vi "LuaVIEW Compile Execute Call.vi"() -> (0 "pass?":bool)   [LabVIEW 2012]
uses:
  typedefs/t_LuaVIEW Reference.ctl
  typedefs/t_LuaVIEW CIN Spinlocked Actions.ctl
  subvis/private/LuaVIEW Pull (string).vi
  subvis/private/LuaVIEW Push (I32).vi
  subvis/private/LuaVIEW Pull (number).vi
  subvis/private/LuaVIEW Push (number).vi
  subvis/private/LuaVIEW Pull (I32).vi
panel:
  in  "script file":path=path "scripts/compile execute call.lua"
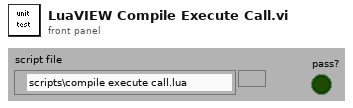
[diagram p1: front panel]
types:
  T1 = enum32{"execute", "initialize", "open_base_state([str:ident])", "open_private_state()", "I32:num=open_states()", "compile(str:name,str:script)", "execute()", "[num:res],...=call(str:function,[num:arg],...)", "[num:res],...=call_required(str:function,I32:required,[num:arg],...)", "close()", "cleanup"}
  T2 = typedef "t_LuaVIEW CIN Spinlocked Actions.ctl" = enum16{"totals", "taskcount", "open", "registerpublic", "registerexport", "revokeexports", "unregnextpublic", "usepublic", "pollexport", "close", "startyieldtest", "endyieldtest", "pollprintbuffer"}
  T3 = typedef "t_LuaVIEW Reference.ctl" = refnum<k1>
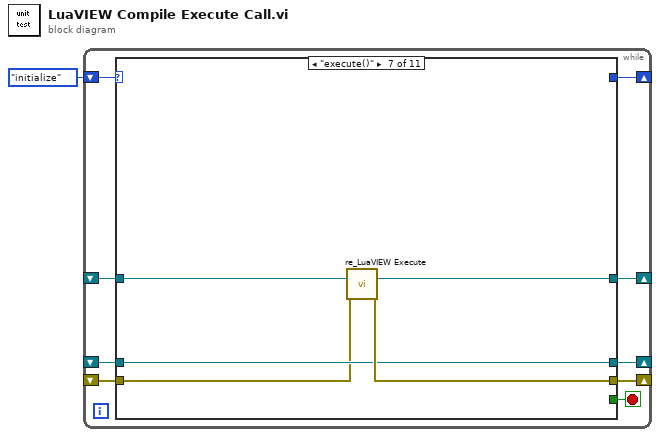
[diagram p0: block diagram]
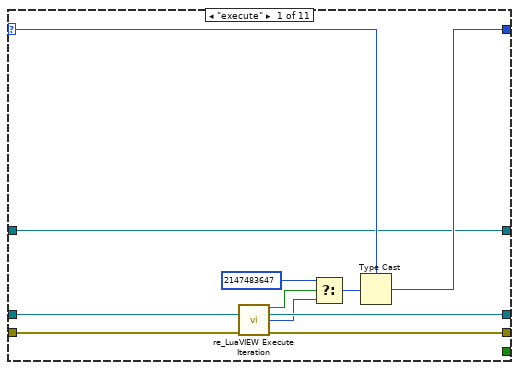
[diagram p2: hidden frame]
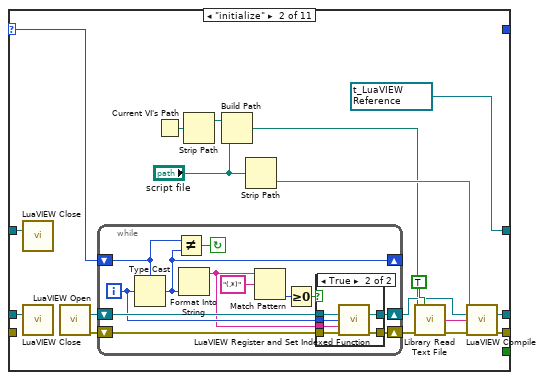
[diagram p3: hidden frame]
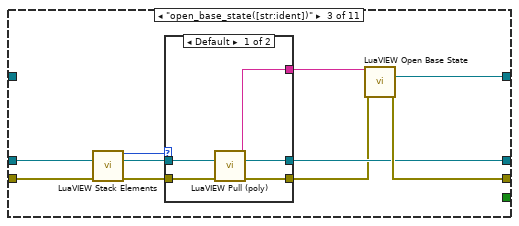
[diagram p5: hidden frame]
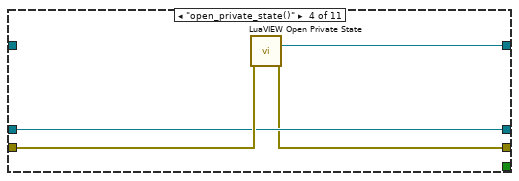
[diagram p7: hidden frame]
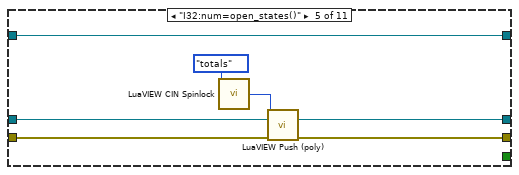
[diagram p8: hidden frame]
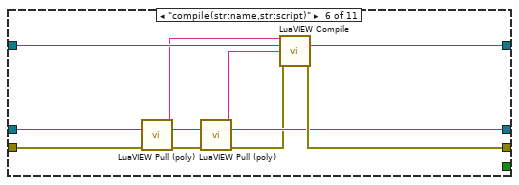
[diagram p9: hidden frame]
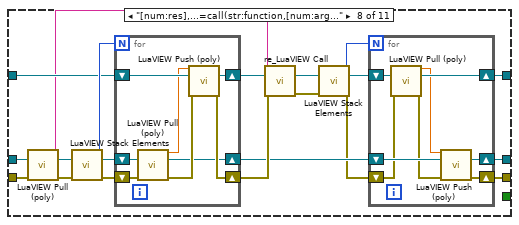
[diagram p10: hidden frame]
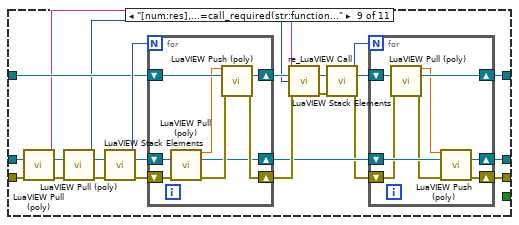
[diagram p11: hidden frame]
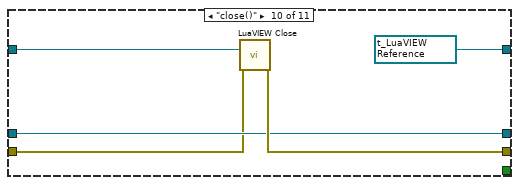
[diagram p12: hidden frame]
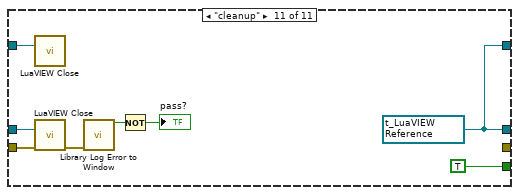
[diagram p13: hidden frame]
diagram:
  n1 = while {
    shift-right: [w8] -> _
    shift-left: T1."initialize" -> [w10]
    shift-right: [w6] -> _
    shift-left: _ -> [w7]
    shift-right: [w5] -> _
    shift-left: _ -> [w4]
    shift-right: [w3] -> _
    shift-left: _ -> [w2]
    stop <- w9 stop-if-true
    n2 = case shown="\"execute()\"" w10 {
      selector: w10 -> [w14 w35 _ _ _ _ _ _ _ _ _]
      tunnel: [_ _ _ _ _ _ _ _ _ _ TRUE] -> w9
      tunnel: [w12 _ _ _ _ _ _ _ _ _ _] -> w8
      tunnel: w7 -> [w21 w39 w66 w79 w81 w91 w100 w115 w156 w181 w191]
      tunnel: [w18 w36 w63 w79 w82 w95 w100 w105 w146 w181 w184] -> w6
      tunnel: [w19 w34 w69 w78 w83 w98 w103 w106 w147 w183 _] -> w5
      tunnel: w4 -> [w20 _ w67 w80 w85 w90 w99 w116 w157 w180 w189]
      tunnel: [w11 w22 w68 w77 w87 w97 w102 w104 w145 w179 w184] -> w3
      tunnel: w2 -> [w11 w23 _ _ w87 w96 w101 w120 w159 w182 w185]
      frame "execute" {
        n3 = call "re_LuaVIEW Execute Iteration.vi"("LuaVIEW reference in"=w21, "init or indexed function error"=w20) -> ("last?"=w16:bool, "LuaVIEW reference out"=w18:T3, "function index"=w17:i32, "final error"=w19:errorcluster)  [unwired: 10 in]
        n4 = Select(t=2147483647, s=w16, f=w17) -> (s? t:f=w13:i32)
        n5 = Type Cast(type=w14, x=w13) -> (*(type *) &x=w12:T1)
      }
      frame "initialize" {
        w22 = T3 refnum items=["LuaVIEW"] ("LuaVIEW reference")
        n6 = call "LuaVIEW Close.vi"("LuaVIEW reference"=w23) -> ()  [unwired: 14 in, 1 out]
        n7 = call "LuaVIEW Close.vi"("LuaVIEW reference"=w39) -> ()  [unwired: 14 in, 1 out]
        n8 = call "LuaVIEW Open.vi"() -> ("LuaVIEW reference"=w37:T3, "error out"=w38:errorcluster)  [unwired: 14 in]
        n9 = while {
          shift-right: [w45] -> w30
          shift-left: w38 -> [w48]
          shift-right: [w46] -> w31
          shift-left: w37 -> [w47]
          shift-right: [w40] -> _
          shift-left: w35 -> [w41]
          i -> [w44]
          stop <- w51 continue-if-true
          n10 = Type Cast(type=w41, x=w44) -> (*(type *) &x=w40:T1)
          n11 = Not Equal?(x=w41, y=w40) -> (x != y?=w51:bool)
          n12 = Format Into String(w40) -> (resulting string=w42:string)  [unwired: 3 in, 1 out]
          n13 = Match Pattern(string=w42, regular expression="(.*)") -> (offset past match=w49:i32)  [unwired: 1 in, 3 out]
          n14 = Greater Or Equal To 0?(x=w49) -> (x >= 0?=w43:bool)
          n15 = case shown="True" w43 {
            tunnel: w47 -> [w53 w56]
            tunnel: w44 -> [_ w57]
            tunnel: w42 -> [_ w54]
            tunnel: [w52 w59] -> w45
            tunnel: [w53 w58] -> w46
            tunnel: w48 -> [w52 w55]
            frame False {
            }
            frame True {
              n16 = call "LuaVIEW Register and Set Indexed Function.vi"("LuaVIEW reference in"=w56, "index"=w57, "synopsis"=w54, "error in (no error)"=w55) -> ("LuaVIEW reference out"=w58:T3, "error out"=w59:errorcluster)  [unwired: 10 in]
            }
          }
        }
        n17 = Current VI's Path() -> (path=w28:path)
        n18 = Strip Path(path=w28) -> (stripped path=w27:path)  [unwired: 1 out]
        n19 = Build Path(base path=w27, name or relative path="script file") -> (appended path=w24:path)
        n20 = Strip Path(path="script file") -> (name=w25:string)  [unwired: 1 out]
        n21 = call "Library Read Text File.vi"("file path"=w24, "convert eol (F)"=TRUE, "error in (no error)"=w30) -> ("read text"=w29:string, "error out"=w32:errorcluster)  [unwired: 10 in, 1 out]
        n22 = call "LuaVIEW Compile.vi"("script name"=w25, "LuaVIEW reference in"=w31, "script"=w29, "error in (no error)"=w32) -> ("LuaVIEW reference out"=w36:T3, "error out"=w34:errorcluster)  [unwired: 10 in]
      }
      frame "open_base_state([str:ident])" {
        n23 = call "LuaVIEW Stack Elements.vi"("LuaVIEW reference in"=w66, "error in (no error)"=w67) -> ("elements"=w65:i32, "LuaVIEW reference out"=w64:T3, "error out"=w62:errorcluster)  [unwired: 11 in]
        n24 = case shown="Default" w65 {
          tunnel: [w71 w76] -> w63
          tunnel: w64 -> [w74 w76]
          tunnel: [w72 w75] -> w61
          tunnel: w62 -> [w73 w75]
          tunnel: [w70 _] -> w60
          frame Default {
            n25 = call-poly "LuaVIEW Pull (poly).vi"("LuaVIEW reference in"=w74, "error in (no error)"=w73) -> ("string"=w70:string, "LuaVIEW reference out"=w71:T3, "error out"=w72:errorcluster)  [unwired: 11 in]
          }
          frame 0 {
          }
        }
        n26 = call "LuaVIEW Open Base State.vi"("close identifier (none)"=w60, "error in (no error)"=w61) -> ("LuaVIEW reference"=w68:T3, "error out"=w69:errorcluster)  [unwired: 12 in]
      }
      frame "open_private_state()" {
        n27 = call "LuaVIEW Open Private State.vi"("error in (no error)"=w80) -> ("LuaVIEW reference"=w77:T3, "error out"=w78:errorcluster)  [unwired: 13 in]
      }
      frame "I32:num=open_states()" {
        n28 = call "LuaVIEW CIN Spinlock.vi"("action"=t_LuaVIEW_CIN_Spinlocked_Actions."totals") -> ("index out"=w84:i32)  [unwired: 8 in, 6 out]
        n29 = call-poly "LuaVIEW Push (poly).vi"("I32"=w84, "LuaVIEW reference in"=w81, "error in (no error)"=w85) -> ("LuaVIEW reference out"=w82:T3, "error out"=w83:errorcluster)  [unwired: 11 in]
      }
      frame "compile(str:name,str:script)" {
        n30 = call-poly "LuaVIEW Pull (poly).vi"("LuaVIEW reference in"=w91, "error in (no error)"=w90) -> ("string"=w88:string, "LuaVIEW reference out"=w93:T3, "error out"=w92:errorcluster)  [unwired: 11 in]
        n31 = call-poly "LuaVIEW Pull (poly).vi"("LuaVIEW reference in"=w93, "error in (no error)"=w92) -> ("string"=w89:string, "LuaVIEW reference out"=w95:T3, "error out"=w94:errorcluster)  [unwired: 11 in]
        n32 = call "LuaVIEW Compile.vi"("script name"=w88, "LuaVIEW reference in"=w96, "script"=w89, "error in (no error)"=w94) -> ("LuaVIEW reference out"=w97:T3, "error out"=w98:errorcluster)  [unwired: 10 in]
      }
      frame "execute()" {
        n33 = call "re_LuaVIEW Execute.vi"("LuaVIEW reference in"=w101, "error in (no error)"=w99) -> ("LuaVIEW reference out"=w102:T3, "error out"=w103:errorcluster)  [unwired: 12 in]
      }
      frame "[num:res],...=call(str:function,[num:arg],...)" {
        n34 = call-poly "LuaVIEW Pull (poly).vi"("LuaVIEW reference in"=w115, "error in (no error)"=w116) -> ("string"=w114:string, "LuaVIEW reference out"=w118:T3, "error out"=w117:errorcluster)  [unwired: 11 in]
        n35 = call "LuaVIEW Stack Elements.vi"("LuaVIEW reference in"=w118, "error in (no error)"=w117) -> ("elements"=w123:i32, "LuaVIEW reference out"=w121:T3, "error out"=w122:errorcluster)  [unwired: 11 in]
        n36 = for {
          N: w123 -> [_]
          shift-right: [w135] -> w113
          shift-left: w122 -> [w138]
          shift-right: [w134] -> w112
          shift-left: w121 -> [w139]
          shift-right: [w133] -> w119
          shift-left: w120 -> [w137]
          n37 = call-poly "LuaVIEW Pull (poly).vi"("LuaVIEW reference in"=w139, "error in (no error)"=w138) -> ("number"=w132:dbl, "LuaVIEW reference out"=w134:T3, "error out"=w136:errorcluster)  [unwired: 11 in]
          n38 = call-poly "LuaVIEW Push (poly).vi"("number"=w132, "LuaVIEW reference in"=w137, "error in (no error)"=w136) -> ("LuaVIEW reference out"=w133:T3, "error out"=w135:errorcluster)  [unwired: 11 in]
        }
        n39 = call "re_LuaVIEW Call.vi"("function name"=w114, "LuaVIEW reference in"=w119, "error in (no error)"=w113) -> ("LuaVIEW reference out"=w108:T3, "error out"=w110:errorcluster)  [unwired: 11 in]
        n40 = call "LuaVIEW Stack Elements.vi"("LuaVIEW reference in"=w108, "error in (no error)"=w110) -> ("elements"=w111:i32, "LuaVIEW reference out"=w107:T3, "error out"=w109:errorcluster)  [unwired: 11 in]
        n41 = for {
          N: w111 -> [_]
          shift-right: [w131] -> w106
          shift-left: w109 -> [w125]
          shift-right: [w130] -> w105
          shift-left: w112 -> [w129]
          shift-right: [w127] -> w104
          shift-left: w107 -> [w128]
          n42 = call-poly "LuaVIEW Pull (poly).vi"("LuaVIEW reference in"=w128, "error in (no error)"=w125) -> ("number"=w126:dbl, "LuaVIEW reference out"=w127:T3, "error out"=w124:errorcluster)  [unwired: 11 in]
          n43 = call-poly "LuaVIEW Push (poly).vi"("number"=w126, "LuaVIEW reference in"=w129, "error in (no error)"=w124) -> ("LuaVIEW reference out"=w130:T3, "error out"=w131:errorcluster)  [unwired: 11 in]
        }
      }
      frame "[num:res],...=call_required(str:function,I32:required,[num:arg],...)" {
        n44 = call-poly "LuaVIEW Pull (poly).vi"("LuaVIEW reference in"=w156, "error in (no error)"=w157) -> ("string"=w155:string, "LuaVIEW reference out"=w141:T3, "error out"=w142:errorcluster)  [unwired: 11 in]
        n45 = call-poly "LuaVIEW Pull (poly).vi"("LuaVIEW reference in"=w141, "error in (no error)"=w142) -> ("I32"=w140:i32, "LuaVIEW reference out"=w144:T3, "error out"=w143:errorcluster)  [unwired: 11 in]
        n46 = call "LuaVIEW Stack Elements.vi"("LuaVIEW reference in"=w144, "error in (no error)"=w143) -> ("elements"=w162:i32, "LuaVIEW reference out"=w160:T3, "error out"=w161:errorcluster)  [unwired: 11 in]
        n47 = for {
          N: w162 -> [_]
          shift-right: [w174] -> w154
          shift-left: w161 -> [w177]
          shift-right: [w173] -> w153
          shift-left: w160 -> [w178]
          shift-right: [w172] -> w158
          shift-left: w159 -> [w176]
          n48 = call-poly "LuaVIEW Pull (poly).vi"("LuaVIEW reference in"=w178, "error in (no error)"=w177) -> ("number"=w171:dbl, "LuaVIEW reference out"=w173:T3, "error out"=w175:errorcluster)  [unwired: 11 in]
          n49 = call-poly "LuaVIEW Push (poly).vi"("number"=w171, "LuaVIEW reference in"=w176, "error in (no error)"=w175) -> ("LuaVIEW reference out"=w172:T3, "error out"=w174:errorcluster)  [unwired: 11 in]
        }
        n50 = call "re_LuaVIEW Call.vi"("function name"=w155, "LuaVIEW reference in"=w158, "required results (no checking needed)"=w140, "error in (no error)"=w154) -> ("LuaVIEW reference out"=w149:T3, "error out"=w151:errorcluster)  [unwired: 10 in]
        n51 = call "LuaVIEW Stack Elements.vi"("LuaVIEW reference in"=w149, "error in (no error)"=w151) -> ("elements"=w152:i32, "LuaVIEW reference out"=w148:T3, "error out"=w150:errorcluster)  [unwired: 11 in]
        n52 = for {
          N: w152 -> [_]
          shift-right: [w170] -> w147
          shift-left: w150 -> [w164]
          shift-right: [w169] -> w146
          shift-left: w153 -> [w168]
          shift-right: [w166] -> w145
          shift-left: w148 -> [w167]
          n53 = call-poly "LuaVIEW Pull (poly).vi"("LuaVIEW reference in"=w167, "error in (no error)"=w164) -> ("number"=w165:dbl, "LuaVIEW reference out"=w166:T3, "error out"=w163:errorcluster)  [unwired: 11 in]
          n54 = call-poly "LuaVIEW Push (poly).vi"("number"=w165, "LuaVIEW reference in"=w168, "error in (no error)"=w163) -> ("LuaVIEW reference out"=w169:T3, "error out"=w170:errorcluster)  [unwired: 11 in]
        }
      }
      frame "close()" {
        w179 = T3 refnum items=["LuaVIEW"] ("LuaVIEW reference")
        n55 = call "LuaVIEW Close.vi"("LuaVIEW reference"=w182, "error in (no error)"=w180) -> ("dup error"=w183:errorcluster)  [unwired: 13 in]
      }
      frame "cleanup" {
        w184 = T3 refnum items=["LuaVIEW"] ("LuaVIEW reference")
        n56 = call "LuaVIEW Close.vi"("LuaVIEW reference"=w185) -> ()  [unwired: 14 in, 1 out]
        n57 = call "LuaVIEW Close.vi"("LuaVIEW reference"=w191, "error in (no error)"=w189) -> ("dup error"=w188:errorcluster)  [unwired: 13 in]
        n58 = call "Library Log Error to Window.vi"("error in (no error)"=w188) -> ("error?"=w187:bool)  [unwired: 13 in, 1 out]
        n59 = Not(x=w187) -> (.not. x?=→"pass?":bool)
      }
    }
  }
